vi "decipher_entity_type.vi"(10 "classpath (fully qualified)":string) -> (2 "entity_type (out)":T1)   [LabVIEW 2016]
uses:
  controls/entity_type.ctl
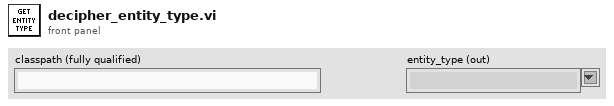
[diagram p1: front panel]
types:
  T1 = typedef "entity_type.ctl" = string
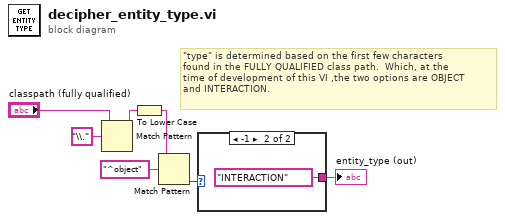
[diagram p0: block diagram]
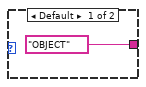
[diagram p2: hidden frame]
diagram:
  # "\"type\" is determined based on the first few characters\nfound in the FULLY QUALIFIED class path.  Which, at the\ntime of development of this VI ,the two options are OBJECT\nand INTERACTION."
  n1 = Match Pattern(string="classpath (fully qualified)", regular expression="\\.") -> (before substring=w6:string)  [unwired: 1 in, 3 out]
  n2 = To Lower Case(string=w6) -> (all lower case string=w5:string)
  n3 = Match Pattern(string=w5, regular expression="^object") -> (offset past match=w3:i32)  [unwired: 1 in, 3 out]
  n4 = case shown="-1" w3 {
    tunnel: [T1 "OBJECT" ("type") T1 "INTERACTION" ("type")] -> w1
    frame Default {
    }
    frame -1 {
    }
  }
  "entity_type (out)" <- w1
